vi "DAC_DC_ouput.vi"() -> ()   [LabVIEW 2010]
uses:
  libdaqVI.lvlib
panel:
  in  "DAC2 电压(V)":dbl
  in  "DAC1 电压(V)":dbl
  in  "DAC2 输出":bool
  out "采集卡状态":bool
  in  "DAC1 输出":bool
  in  "退出程序":bool
  out "设备名称":string
  out "设备数量":u32
  # "范例说明：\n1、支持的采集卡：DAQ-USB3212、DAQ-USB3213、DAQ-USB3214\nDAQ-USB3212 量程:0-5V\nDAQ-USB3213 量程:0-10V\nDAQ-USB3214 量程:±10V\n2、运行程序之后，在电压输入框中输入电压值，再点击“DAC输出”，超过量程的电压值将会被截断；"
  # "DAQ-DAC直流输出演示程序"
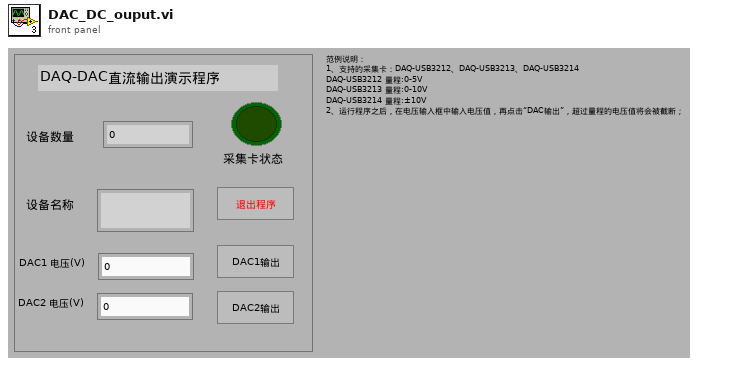
[diagram p1: front panel]
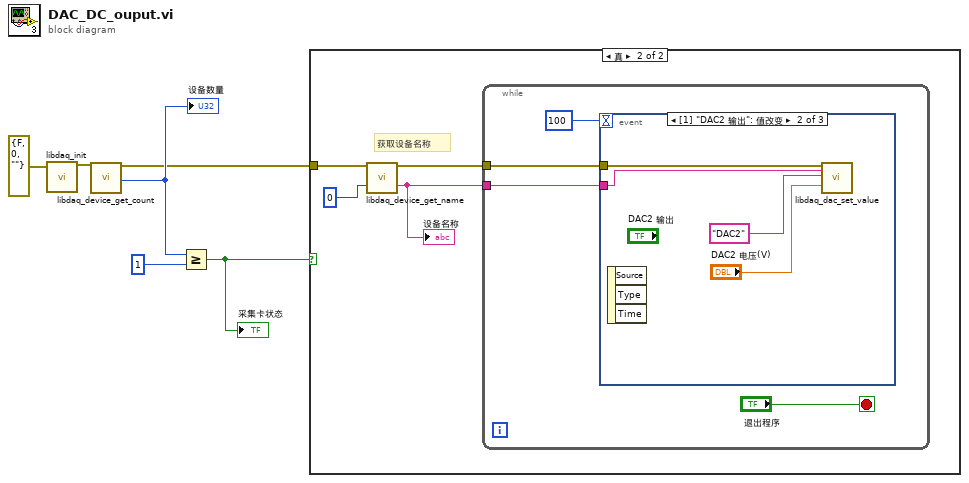
[diagram p0: block diagram]
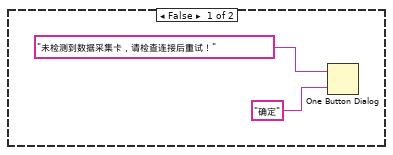
[diagram p2: hidden frame]
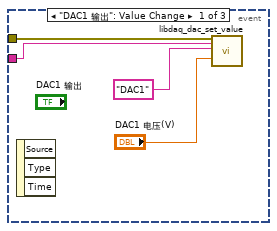
[diagram p3: hidden frame]
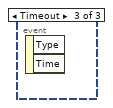
[diagram p4: hidden frame]
diagram:
  n1 = call "libdaq_init.vi"("error in (no error)"=errorcluster {"status"=FALSE, "code"=0, "source"=""}) -> ("error out"=w3:errorcluster)  [unwired: 18 in]
  n2 = call "libdaq_device_get_count.vi"("error in (no error)"=w3) -> ("error out"=w1:errorcluster, "device_count"=w2:i32)  [unwired: 17 in]
  "设备数量" <- w2
  n3 = Greater Or Equal?(x=w2, y=u32 1 ("name length")) -> (x >= y?=w5:bool)
  "采集卡状态" <- w5
  n4 = case shown="真" w5 {
    tunnel: w1 -> [_ w12]
    frame False {
      n5 = One Button Dialog(message="未检测到数据采集卡，请检查连接后重试！" ("消息"), button name ("OK")="确定" ("按钮名称（“确定”）")) -> ()  [unwired: 1 out]
    }
    frame True {
      # "获取设备名称"
      n6 = call "libdaq_device_get_name.vi"("error in (no error)"=w12, "device_index"=u32 0 ("name length")) -> ("error out"=w11:errorcluster, "device_name"=w9:string)  [unwired: 16 in]
      "设备名称" <- w9
      n7 = while {
        tunnel: w11 -> [w14]
        tunnel: w9 -> [w13]
        stop <- "退出程序" stop-if-true
        n8 = event shown="[1] \"DAC2 输出\": 值改变" {
          selector: _ -> [_ _ _]
          dyn-events: _ -> [_ _ _]
          timeout: 100 -> [_ _ _]
          tunnel: w13 -> [w19 w23 _]
          tunnel: w14 -> [w20 w24 _]
          event "DAC1 输出": Value Change {
            n9 = event-data() -> ()  [unwired: 1 in, 3 out]
            n10 = call "libdaq_dac_set_value.vi"("error in (no error)"=w20, "device_name"=w19, "module_name"="DAC1", "value"="DAC1 电压(V)") -> ()  [unwired: 13 in, 3 out]
          }
          event "DAC2 输出": Value Change {
            n11 = event-data() -> ()  [unwired: 1 in, 3 out]
            n12 = call "libdaq_dac_set_value.vi"("error in (no error)"=w24, "device_name"=w23, "module_name"="DAC2", "value"="DAC2 电压(V)") -> ()  [unwired: 13 in, 3 out]
          }
          event Timeout {
            n13 = event-data() -> ()  [unwired: 1 in, 2 out]
          }
        }
      }
    }
  }
